vi "zmq_poll_array.vi"(4 "error in":errorcluster, 5 "timeout":i32, 6 "poll type":T1[](array[typedef]), 7 "sockets":refnum<class "zmq_socket.lvclass">[](array[class])) -> (0 "error out":errorcluster, 1 "timed out?":bool, 2 "nevents":u32, 3 "polled events":T1[](array[typedef]))   [LabVIEW 2019, in "zeromq.lvlib" / "zmq_socket.lvclass"]
doc: "Poll multiple sockets and for events. Blocks for <b>timeout</b> milliseconds or until an event occur on any of the given <b>sockets</b>. If no event happens, then <b>timed out?</b> is True.\n\nThe array <b>poll type</b> contains events to look for, and <b>must</b> contain a value for each socket provided. The enumeration contains the events to poll for.\n\nIf <b>timeout</b> is zero, the function returns immediately, regardless of whether any events are waiting. If <b>timeout</b> is negative, the function will block until an event occurs.\n\nWhile the call is blocking, the sockets cannot be used for another blocking operation. If a termination event occurs while blocking, the blocked sockets are closed.\n\nDetailed API documentation: http://api.zeromq.org/3-2:zmq-poll"
uses:
  zmq_socket.lvclass
  poll_type.ctl
  zmq_socket.lvclass/zmq_socket.ctl
  <vilib>/Utility/error.llb/Error Cluster From Error Code.vi
  zeromq.lvlib
panel:
  # "ØMQ"
  # "labview"
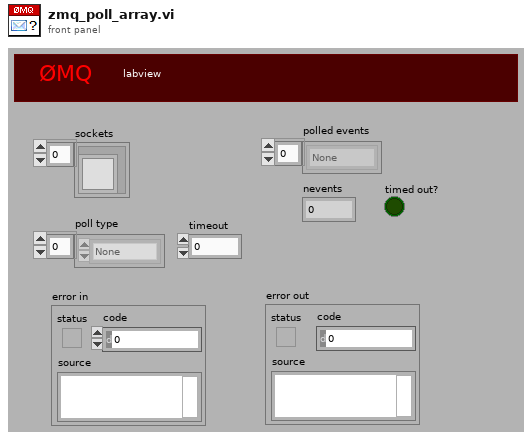
[diagram p1: front panel]
types:
  T1 = typedef "zeromq.lvlib/poll_type.ctl" = enum16{"None", "In", "Out", "In/Out"}
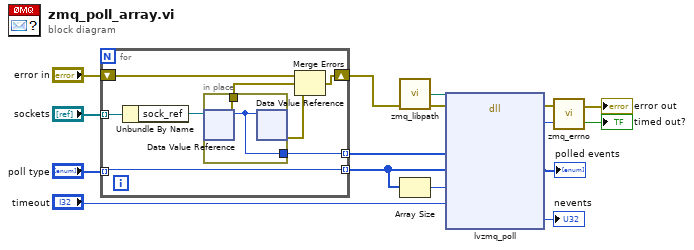
[diagram p0: block diagram]
diagram:
  n1 = for {
    tunnel: "sockets" -> [w23] mode=indexing
    tunnel: [w21] -> w8 mode=indexing
    tunnel: [w22] -> w5 mode=indexing
    tunnel: "poll type" -> [w22] mode=indexing
    shift-right: [w16] -> w1
    shift-left: "error in" -> [w19]
    n2 = Unbundle By Name(w23) -> ("sock_ref"=w20:refnum<data-value>)
    n3 = in-place {
      in-place-border: [w25] -> w21
      in-place-border: [w24] -> w18
      n4 = in-place-dvr #1(w20) -> (w25:u64, w24:errorcluster)
      n5 = in-place-dvr #1(w25) -> (w17:errorcluster)  [unwired: 1 out]
    }
    n6 = Merge Errors(w19, w18, w17) -> (w16:errorcluster)
  }
  n7 = call "zmq_libpath.vi"() -> ("path"=w3:path)
  n8 = Array Size(array=w5) -> (size(s)=w4:i32)
  n9 = dll-call lib="?" fn="lvzmq_poll" ("zmq_labview.dll:lvzmq_socket")(path in=w3, error in=w1, "socket"=w8, "evt"=w5, "n"=w4, "timeout"="timeout") -> (error out=w15:errorcluster, "return type"=w14:i32, "evt"=→"polled events":i32[], "nevents"=→"nevents":u32)  [unwired: 7 in, 1 out]
  n10 = call "zmq_errno.vi"("retval"=w14, "error in"=w15) -> ("again?"=→"timed out?":bool, "error out"=→"error out":errorcluster)
